vi "Polling Core.vi"(8 "Error In":errorcluster, 11 "Beep in":refnum<class "Beep.lvclass">) -> (0 "Error Out":errorcluster, 3 "Beep out":refnum<class "Beep.lvclass">)   [LabVIEW 2016, in "CS++BeepActor.lvlib" / "Beep.lvclass"]
doc: "Implement the pseudo-periodic action in your override.vi."
uses:
  Beep.lvclass
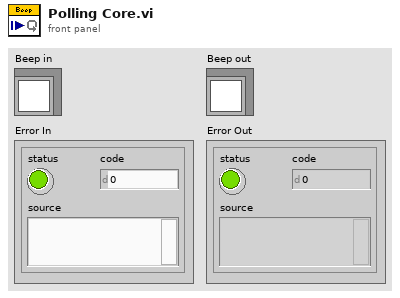
[diagram p1: front panel]
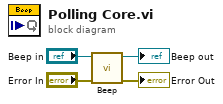
[diagram p0: block diagram]
diagram:
  n1 = call "Beep.vi"("error in (no error)"="Error In", "Beep in"="Beep in") -> ("error out"=→"Error Out":errorcluster, "Beep out"=→"Beep out":refnum<class "Beep.lvclass">)  [unwired: 8 in]
